vi "Image_Save_Handler.vi"(8 "Stop?":bool, 9 "Data":T3={"L16 Linear Actuator"="", "XE 1000 Pump"="", "Camera1"="", "Camera2"="", "Img_Capt"=FALSE, "Actuator"=FALSE, "Pump"=FALSE, "Cam 1"=FALSE, "Cam 2"=FALSE, "Empty_Refill"=FALSE, "Crop"=FALSE, "Light intensity"=100, "Exposure Time"=1000.0, "Sample Name"="Test Sample", "Operator"="MRJ", "Calibration 1"=path "C:/Users/au540322/Desktop/IHS_Project/images/Debris/Debris_0/Debris_0_2019_06_01-23-32-49-686.PNG", "Calibration 2"=path "C:/Users/au540322/Desktop/IHS_Project/images/Debris/Debris_0/Debris_0_2019_06_01-23-32-49-686.PNG", "Framerate"=1, "Timeout Sample"=0, "Collection date"="MRJ", "Sample size threshold"=1, "Empty start"=1, "Command"="MRJ", "Station"="", "Species Name"="", "Other Notes"="", "Aperture"=enum."Item 0", "Image Process Queue Size"=500, "Image Save Queue Size"=500, "Overload threshold"=500, "Max Framerate"=100, "Rectangle 1"={"Left"=0, "Top"=0, "Right"=0, "Bottom"=0, "Rotation"=0.0}, "Rectangle 2"={"Left"=0, "Top"=0, "Right"=0, "Bottom"=0, "Rotation"=0.0}, "Detection Region %"=0.0, "Detect 1"=path "C:/Users/au540322/Desktop/IHS_Project/images/Debris/Debris_0/Debris_0_2019_06_01-23-32-49-686.PNG", "Detect 2"=path "C:/Users/au540322/Desktop/IHS_Project/images/Debris/Debris_0/Debris_0_2019_06_01-23-32-49-686.PNG", "Max large object threshold"=0, "Open(T)/Close(F)"=FALSE, "Img_Capt Begin"=FALSE, "Dispense Speed"=100, "Flush Size"=100, "Location"="Station", "Latitude"="Station", "Longitude"="Station", "Determiner"="Station", "Sex"="Station", "Camera1_Img"=refnum, "Camera2_Img"=refnum, "Img1_Orig_Disp"=refnum, "Img2_Orig_Disp"=refnum, "Img1_Orig_RGB"=refnum, "Img2_Orig_RGB"=refnum, "Blue_Plane_Extract"=refnum, "Subtracted_Plane"=refnum, "Img1_Binary"=refnum, "Img2_Binary"=refnum, "Crop_Mask"=refnum, "Img1_Save"=refnum, "Img2_Save"=refnum, "Img1_Cali_Full"=refnum, "Img2_Cali_Full"=refnum, "Img1_Cali_Detect"=refnum, "Img2_Cali_Detect"=refnum, "Cam 1 queue"=refnum, "Cam 2 queue"=refnum, "Cam 1 - save queue"=refnum, "Cam 2 - save queue"=refnum} {"Flush Size" min=1; "Dispense Speed" min=1; "Rectangle 2"."Rotation" format="%.2f"; "Rectangle 2"."Left" scale=0.0..1024.0; "Rectangle 2"."Right" scale=0.0..1024.0; "Rectangle 1"."Rotation" format="%.2f"; "Rectangle 1"."Left" scale=0.0..1024.0; "Rectangle 1"."Right" scale=0.0..1024.0; "Max Framerate" min=1; "Overload threshold" min=1; "Image Save Queue Size" min=1; "Image Process Queue Size" min=1; "Empty start" min=1; "Sample size threshold" min=1; "Framerate" min=1; "Light intensity" scale=0.0..100.0}, 11 "first iteration":bool) -> (0 "Stop out":bool, 1 "max queue":i32, 2 "timeout":bool, 3 "Queue size":T2, 5 "Image Save 2":T1, 7 "Image Save 1":T1)   [LabVIEW 2020]
doc: "Saves image files from cameras in specified folder location."
uses:
  controls/Data.ctl
  <vilib>/userDefined/High Color/IMAQdx.ctl
  <vilib>/vision/Image Controls.llb/IMAQ Image.ctl
  Camera_ID.ctl
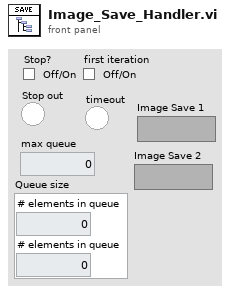
[diagram p1: front panel]
types:
  T1 = typedef "IMAQ Image.ctl" = refnum<image>
  T2 = cluster{"# elements in queue":i32, "# elements in queue":i32}
  T3 = typedef "Data.ctl" = cluster{"L16 Linear Actuator":refnum<visa-resource-name>, "XE 1000 Pump":refnum<visa-resource-name>, "Camera1":T4, "Camera2":T4, "Img_Capt":bool, "Actuator":bool, "Pump":bool, "Cam 1":bool, "Cam 2":bool, "Empty_Refill":bool, "Crop":bool, "Light intensity":i32, "Exposure Time":dbl, "Sample Name":string, "Operator":string, "Calibration 1":path, "Calibration 2":path, "Framerate":i32, "Timeout Sample":i32, "Collection date":string, "Sample size threshold":i32, "Empty start":u32, "Command":string, "Station":string, "Species Name":string, "Other Notes":string, "Aperture":enum32{"Item 0", "Item 1", "Item 2", "Item 3"}, "Image Process Queue Size":i32, "Image Save Queue Size":i32, "Overload threshold":i32, "Max Framerate":i32, "Rectangle 1":T5, "Rectangle 2":T5, "Detection Region %":dbl, "Detect 1":path, "Detect 2":path, "Max large object threshold":i32, "Open(T)/Close(F)":bool, "Img_Capt Begin":bool, "Dispense Speed":i32, "Flush Size":i32, "Location":string, "Latitude":string, "Longitude":string, "Determiner":string, "Sex":string, "Camera1_Img":T1, "Camera2_Img":T1, "Img1_Orig_Disp":T1, "Img2_Orig_Disp":T1, "Img1_Orig_RGB":T1, "Img2_Orig_RGB":T1, "Blue_Plane_Extract":T1, "Subtracted_Plane":T1, "Img1_Binary":T1, "Img2_Binary":T1, "Crop_Mask":T1, "Img1_Save":T1, "Img2_Save":T1, "Img1_Cali_Full":T1, "Img2_Cali_Full":T1, "Img1_Cali_Detect":T1, "Img2_Cali_Detect":T1, "Cam 1 queue":refnum<queue>, "Cam 2 queue":refnum<queue>, "Cam 1 - save queue":refnum<queue>, "Cam 2 - save queue":refnum<queue>}
  T4 = typedef "IMAQdx.ctl" = refnum<k21>
  T5 = typedef "IMAQ Rectangle" = cluster{"Left":i32, "Top":i32, "Right":i32, "Bottom":i32, "Rotation":dbl}
  T6 = typedef "Camera_ID.ctl" = enum16{"Camera 1", "Camera 2"}
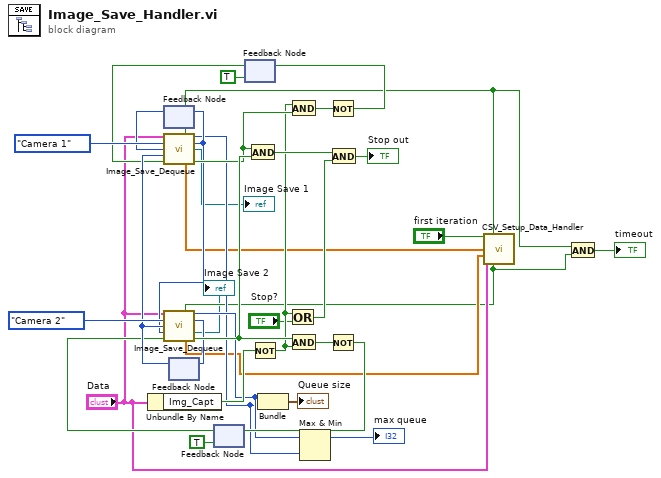
[diagram p0: block diagram]
diagram:
  n1 = Unbundle By Name("Data") -> ("Img_Capt"=w30:bool)
  n2 = feedback #1() -> (w23:i32)  [unwired: 1 in]
  n3 = feedback #2() -> (w21:i32)  [unwired: 1 in]
  n4 = feedback #3(TRUE) -> (w16:bool)
  n5 = feedback #4(TRUE) -> (w18:bool)
  n6 = call "Image_Save_Dequeue.vi"("Data"="Data", "Camera"=Camera_ID."Camera 1", "Old"=w23, "Other"=w21, "Queue active"=w18) -> ("timed out?"=w6:bool, "# elements in queue"=w11:i32, "State out"=w20:i32, "Image Save 1"=→"Image Save 1":T1, "Sample Data"=w9:dbl[], "Last image"=w27:bool)  [unwired: 4 in, 1 out]
  n7 = feedback-in #1(w20) -> ()
  n8 = call "Image_Save_Dequeue.vi"("Data"="Data", "Camera"=Camera_ID."Camera 2", "Old"=w21, "Other"=w20, "Queue active"=w16) -> ("timed out?"=w5:bool, "# elements in queue"=w12:i32, "State out"=w22:i32, "Image Save 2"=→"Image Save 2":T1, "Sample Data"=w8:dbl[], "Last image"=w29:bool)  [unwired: 4 in, 1 out]
  n9 = feedback-in #2(w22) -> ()
  n10 = And(x=w27, y=w29) -> (x .and. y?=w33:bool)
  n11 = Not(x=w30) -> (.not. x?=w26:bool)
  n12 = Bundle("# elements in queue"=w12, "# elements in queue"=w11) -> (→"Queue size":T2)  [unwired: 1 in]
  n13 = Or(x=w26, y="Stop?") -> (x .or. y?=w31:bool)
  n14 = And(x=w26, y=w27) -> (x .and. y?=w25:bool)
  n15 = And(x=w29, y=w26) -> (x .and. y?=w28:bool)
  n16 = Max & Min(x=w12, y=w11) -> (max(x,y)=→"max queue":i32)  [unwired: 1 out]
  n17 = Not(x=w25) -> (.not. x?=w19:bool)
  n18 = feedback-in #4(w19) -> ()
  n19 = Not(x=w28) -> (.not. x?=w17:bool)
  n20 = feedback-in #3(w17) -> ()
  n21 = And(x=w33, y=w31) -> (x .and. y?=→"Stop out":bool)
  n22 = call "CSV_Setup_Data_Handler.vi"("first iteration"="first iteration", "Timeout 1"=w6, "Sample Data"=w9, "Sample Data 2"=w8, "Data"="Data", "Timeout 2"=w5) -> ()  [unwired: 10 in]
  n23 = And(x=w6, y=w5) -> (x .and. y?=→"timeout":bool)
